vi "clLabview_BDPW_calc.vi"(0 "vi_lib.lvlib:clLabview.lvclass":refnum<class "clLabview.lvclass">, 2 "new Password":string="LVSR") -> (14 "MD5 password":string, 15 "Hash 1":string, 16 "Hash 2":string, 17 "MD5 password (Hex)":string, 18 "Hash 1 (Hex)":string, 19 "Hash 2 (Hex)":string)   [LabVIEW 2016, in "vi_lib.lvlib" / "clLabview.lvclass"]
uses:
  clLabview.lvclass
  clLabview.lvclass/clLabview.ctl
  vi_lib.lvlib
  clFileReader/clFileReader.lvclass
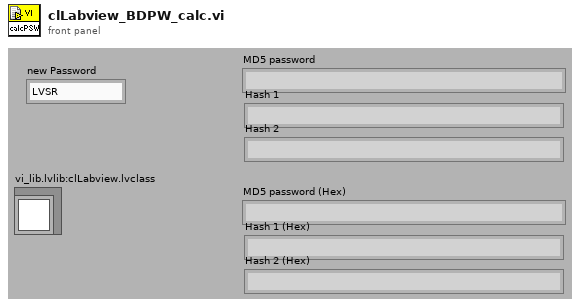
[diagram p1: front panel]
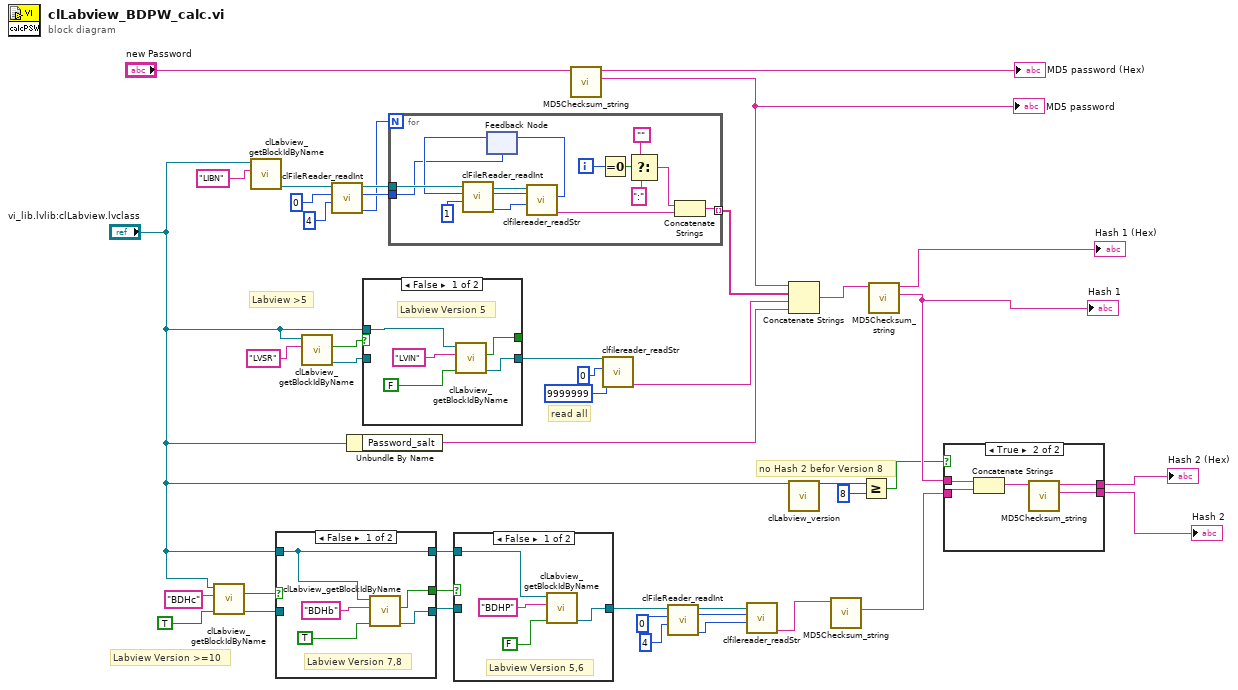
[diagram p0: block diagram]
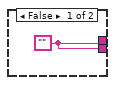
[diagram p2: hidden frame]
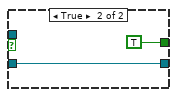
[diagram p3: hidden frame]
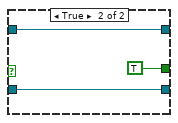
[diagram p5: hidden frame]
diagram:
  # "no Hash 2 befor Version 8"
  # "read all"
  # "Labview >5"
  # "Labview Version >=10"
  n1 = call "clLabview_getBlockIdByName.vi"("use compression (off)"=TRUE, "Block Name"="BDHc", "vi_lib.lvlib:clLabview.lvclass"="vi_lib.lvlib:clLabview.lvclass") -> ("Block Content"=w30:refnum<class "clFileReader.lvclass">, "Name found?"=w32:bool)  [unwired: 1 in, 5 out]
  n2 = call "clLabview_getBlockIdByName.vi"("Block Name"="LIBN", "vi_lib.lvlib:clLabview.lvclass"="vi_lib.lvlib:clLabview.lvclass") -> ("Block Content"=w39:refnum<class "clFileReader.lvclass">)  [unwired: 2 in, 6 out]
  n3 = case shown="False" w32 {
    tunnel: "vi_lib.lvlib:clLabview.lvclass" -> [w44 w49]
    tunnel: w30 -> [_ w51]
    tunnel: [w47 w51] -> w15
    tunnel: [w45 TRUE ("Name found?")] -> w14
    tunnel: [w44 w49] -> w6
    frame False {
      # "Labview Version 7,8"
      n4 = call "clLabview_getBlockIdByName.vi"("use compression (off)"=TRUE, "Block Name"="BDHb", "vi_lib.lvlib:clLabview.lvclass"=w44) -> ("Block Content"=w47:refnum<class "clFileReader.lvclass">, "Name found?"=w45:bool)  [unwired: 1 in, 5 out]
    }
    frame True {
    }
  }
  n5 = call "clLabview_getBlockIdByName.vi"("Block Name"="LVSR", "vi_lib.lvlib:clLabview.lvclass"="vi_lib.lvlib:clLabview.lvclass") -> ("Block Content"=w11:refnum<class "clFileReader.lvclass">, "Name found?"=w13:bool)  [unwired: 2 in, 5 out]
  n6 = call "clFileReader_readInt.vi"("size"=u32 4, "offset"=u32 0, "clFileReader.lvclass IN"=w39) -> ("OUT Value"=w7:u32, "new offset"=w9:u32, "clFileReader.lvclass OUT"=w10:refnum<class "clFileReader.lvclass">)  [unwired: 6 out]
  n7 = Unbundle By Name("vi_lib.lvlib:clLabview.lvclass") -> ("Password_salt"=w17:string)
  n8 = case shown="False" w13 {
    tunnel: "vi_lib.lvlib:clLabview.lvclass" -> [w56 _]
    tunnel: w11 -> [_ w58]
    tunnel: [w54 w58] -> w12
    tunnel: [w52 TRUE ("Name found?")] -> _
    frame False {
      # "Labview Version 5"
      n9 = call "clLabview_getBlockIdByName.vi"("use compression (off)"=FALSE, "Block Name"="LVIN", "vi_lib.lvlib:clLabview.lvclass"=w56) -> ("Block Content"=w54:refnum<class "clFileReader.lvclass">, "Name found?"=w52:bool)  [unwired: 1 in, 5 out]
    }
    frame True {
    }
  }
  n10 = for {
    N: w7 -> [_]
    tunnel: w10 -> [w73]
    tunnel: w9 -> [w66]
    tunnel: [w64] -> w8 mode=indexing
    i -> [w63]
    n11 = feedback #1(w66) -> (w67:u32)
    n12 = call "clFileReader_readInt.vi"("size"=u32 1, "offset"=w67, "clFileReader.lvclass IN"=w73) -> ("OUT Value"=w69:u32, "new offset"=w70:u32, "clFileReader.lvclass OUT"=w71:refnum<class "clFileReader.lvclass">)  [unwired: 6 out]
    n13 = call "clfilereader_readStr.vi"("size"=w69, "offset"=w70, "clFileReader.lvclass IN"=w71) -> ("ReadStr - OUT Value"=w65:string, "new offset"=w68:u32)  [unwired: 7 out]
    n14 = feedback-in #1(w68) -> ()
    n15 = Equal To 0?(x=w63) -> (x = 0?=w62:bool)
    n16 = Select(t="", s=w62, f=":" ("ReadStr - OUT Value")) -> (s? t:f=w61:string)
    n17 = Concatenate Strings(w61, w65) -> (w64:string)
  }
  n18 = case shown="False" w14 {
    tunnel: w15 -> [_ w78]
    tunnel: [w76 w78] -> w16
    tunnel: w6 -> [w74 _]
    frame False {
      # "Labview Version 5,6"
      n19 = call "clLabview_getBlockIdByName.vi"("use compression (off)"=FALSE, "Block Name"="BDHP", "vi_lib.lvlib:clLabview.lvclass"=w74) -> ("Block Content"=w76:refnum<class "clFileReader.lvclass">)  [unwired: 1 in, 6 out]
    }
    frame True {
    }
  }
  n20 = call "MD5Checksum_string.vi"("Message String"="new Password") -> ("MD5 message-digest (Ascii)"=w19:string, "MD5 message-digest (Hex)"=→"MD5 password (Hex)":string)  [unwired: 9 out]
  "MD5 password" <- w19
  n21 = call "clfilereader_readStr.vi"("size"=u32 9999999, "offset"=u32 0, "clFileReader.lvclass IN"=w12) -> ("ReadStr - OUT Value"=w1:string)  [unwired: 8 out]
  n22 = call "clFileReader_readInt.vi"("size"=u32 4, "offset"=u32 0, "clFileReader.lvclass IN"=w16) -> ("OUT Value"=w24:u32, "new offset"=w25:u32, "clFileReader.lvclass OUT"=w26:refnum<class "clFileReader.lvclass">)  [unwired: 6 out]
  n23 = call "clfilereader_readStr.vi"("size"=w24, "offset"=w25, "clFileReader.lvclass IN"=w26) -> ("ReadStr - OUT Value"=w23:string)  [unwired: 8 out]
  n24 = Concatenate Strings(w19, w8, w1, w17) -> (w34:string)
  n25 = call "clLabview_version.vi"("vi_lib.lvlib:clLabview.lvclass"="vi_lib.lvlib:clLabview.lvclass") -> ("major"=w4:u8)  [unwired: 18 out]
  n26 = call "MD5Checksum_string.vi"("Message String"=w23) -> ("MD5 message-digest (Ascii)"=w21:string)  [unwired: 10 out]
  n27 = Greater Or Equal?(x=w4, y=u8 8) -> (x >= y?=w2:bool)
  n28 = call "MD5Checksum_string.vi"("Message String"=w34) -> ("MD5 message-digest (Ascii)"=w20:string, "MD5 message-digest (Hex)"=→"Hash 1 (Hex)":string)  [unwired: 9 out]
  "Hash 1" <- w20
  n29 = case shown="True" w2 {
    tunnel: [w79 w84] -> w22
    tunnel: w21 -> [_ w83]
    tunnel: w20 -> [_ w81]
    tunnel: [w79 w80] -> w18
    frame False {
      w79 = "" ("MD5 message-digest (Hex)")
    }
    frame True {
      n30 = Concatenate Strings(w81, w83) -> (w82:string)
      n31 = call "MD5Checksum_string.vi"("Message String"=w82) -> ("MD5 message-digest (Ascii)"=w80:string, "MD5 message-digest (Hex)"=w84:string)  [unwired: 9 out]
    }
  }
  "Hash 2 (Hex)" <- w22
  "Hash 2" <- w18
